vi "Save Transport TDMS File.vi"(6 "append?":bool, 8 "error in (no error)":errorcluster, 11 "Control Experiment in":refnum<class "Control Experiment.lvclass">) -> (0 "error out":errorcluster, 3 "Control Experiment out":refnum<class "Control Experiment.lvclass">)   [LabVIEW 2019, in "Control Experiment.lvclass"]
uses:
  Control Experiment.lvclass
  <userlib>/LevyLab/LV-Data/LV-Data.TDMS/LV-Data.TDMS.lvclass
  Control Experiment.lvclass/Control Experiment.ctl
  <userlib>/LevyLab/LV-Data/LV-Data/Typedefs/Operation--enum.ctl
  0a851934-036a-4f78-963b-fa5fb1e10b30.vi
  <userlib>/LevyLab/LV-Data/LV-Data/Typedefs/File Type--enum.ctl
  <userlib>/LevyLab/LV-Data/LV-Data/LV-Data.lvclass
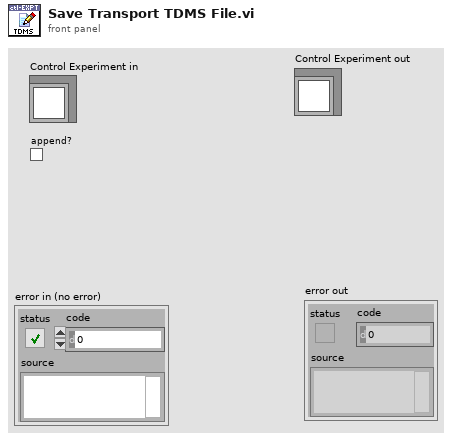
[diagram p1: front panel]
types:
  T1 = typedef "LV-Data.lvclass/File Type--enum.ctl" = enum16{"DAT", "ITX", "TDMS", "VI"}
  T2 = typedef "LV-Data.lvclass/Operation--enum.ctl" = enum16{"Read", "Write", "Write + Append"}
  T3 = typedef "LV-Data.lvclass/Dictionary--cluster.ctl" = cluster{"key":string, "value":variant}
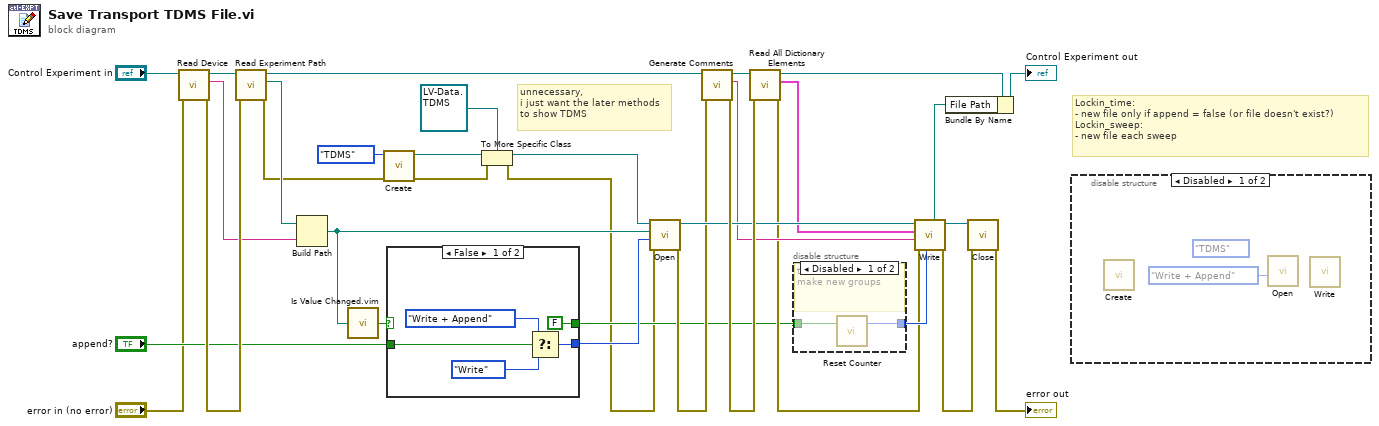
[diagram p0: block diagram]
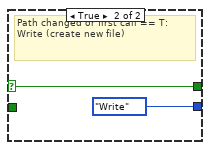
[diagram p2: hidden frame]
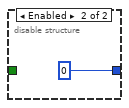
[diagram p4: hidden frame]
diagram:
  # "unnecessary,\ni just want the later methods\nto show TDMS"
  # "Lockin_time:\n- new file only if append = false (or file doesn't exist?)\nLockin_sweep:\n- new file each sweep"
  n1 = call "Read Device.vi"("error in (no error)"="error in (no error)", "Control Experiment in"="Control Experiment in") -> ("error out"=w32:errorcluster, "Device"=w25:string, "Control Experiment out"=w33:refnum<class "Control Experiment.lvclass">)  [unwired: 7 in]
  n2 = call "Read Experiment Path.vi"("error in (no error)"=w32, "Control Experiment in"=w33) -> ("error out"=w2:errorcluster, "Experiment Path"=w24:path, "Control Experiment out"=w15:refnum<class "Control Experiment.lvclass">)  [unwired: 7 in]
  n3 = Build Path(base path=w24, name or relative path=w25) -> (appended path=w21:path)
  n4 = call "Is Value Changed.vim"("value"=w21) -> ("changed or first call?"=w10:bool)
  n5 = call <userlib>:"Create.vi"("error in (no error)"=w2, "File Type"=File_Type--enum."TDMS") -> ("error out"=w3:errorcluster, "Data out"=w5:refnum<class "LV-Data.lvclass">)  [unwired: 8 in]
  n6 = case shown="False" w10 {
    selector: w10 -> [_ w39]
    tunnel: "append?" -> [w38 _]
    tunnel: [w35 Operation--enum."Write" ("Operation")] -> w9
    tunnel: [FALSE w39] -> w8
    frame False {
      n7 = Select(t=Operation--enum."Write + Append" ("Operation"), s=w38, f=Operation--enum."Write" ("Operation")) -> (s? t:f=w35:T2)
    }
    frame True {
      # "Path changed or first call == T:\nWrite (create new file)"
    }
  }
  n8 = To More Specific Class(target class=refnum<class "LV-Data.TDMS.lvclass"> refnum ("Data.TDMS in"), reference=w5, error in=w3) -> (specific class reference=w4:refnum<class "LV-Data.TDMS.lvclass">, error out=w1:errorcluster)
  n9 = call-dynamic "Open.vi"("error in (no error)"=w1, "Operation"=w9, "Path"=w21, "Data.TDMS in"=w4) -> ("error out"=w12:errorcluster, "Data.TDMS out"=w28:refnum<class "LV-Data.TDMS.lvclass">)  [unwired: 6 in]
  n10 = call "Generate Comments.vi"("error in (no error)"=w12, "Control Experiment"=w15) -> ("error out"=w30:errorcluster, "Comments"=w18:string, "Control Experiment out"=w31:refnum<class "Control Experiment.lvclass">)  [unwired: 6 in]
  n11 = call "Read All Dictionary Elements.vi"("error in (no error)"=w30, "Control Experiment in"=w31) -> ("error out"=w11:errorcluster, "Items"=w13:T3[], "Control Experiment out"=w14:refnum<class "Control Experiment.lvclass">)  [unwired: 7 in]
  n12 = disable-structure shown="Disabled" {
    disable-tunnel: [w42 0 ("Append Index")] -> w19
    disable-tunnel: w8 -> [w41 _]
    frame Disabled {
      # "this counter will make new groups"
      n13 = call "Reset Counter.vi"("Reset"=w41) -> ("Counter"=w42:i32)  [unwired: 2 in]
    }
    frame Enabled {
    }
  }
  n14 = call-dynamic "Write.vi"("Append Index"=w19, "error in (no error)"=w11, "Notes"=w18, "Data (Dictionary)"=w13, "Data.TDMS in"=w28) -> ("error out"=w27:errorcluster, "Data.TDMS out"=w26:refnum<class "LV-Data.TDMS.lvclass">, "Path out"=w22:path)  [unwired: 4 in]
  n15 = Bundle By Name(cluster=w14, "File Path"=w22) -> (→"Control Experiment out":refnum<class "Control Experiment.lvclass">)
  n16 = call-dynamic "Close.vi"("error in (no error)"=w27, "Data.TDMS in"=w26) -> ("error out"=→"error out":errorcluster)  [unwired: 8 in, 1 out]
  n17 = disable-structure shown="Disabled" {
    frame Disabled {
      (unwired) File_Type--enum."TDMS" ("File Type")
      n18 = call <userlib>:"Create.vi"() -> ()  [unwired: 10 in, 2 out]
      n19 = call-dynamic "Open.vi"("Operation"=Operation--enum."Write + Append") -> ()  [unwired: 9 in, 2 out]
      n20 = call-dynamic "Write.vi"() -> ()  [unwired: 9 in, 3 out]
    }
    frame Enabled {
    }
  }
